vi "GetObjectID.vi"(0 "reference in":refnum<class "G#RemoteProxy.lvclass">, 5 "error in (no error)":errorcluster) -> (14 "reference out":refnum<class "G#RemoteProxy.lvclass">, 15 "object ID":u32 format="%x", 19 "error out":errorcluster)   [LabVIEW 2017, in "G#RemoteProxy.lvclass"]
doc: "Returns the unique object ID for the specified object."
uses:
  G#RemoteProxy.lvclass
  G#Object/G#Object.lvclass
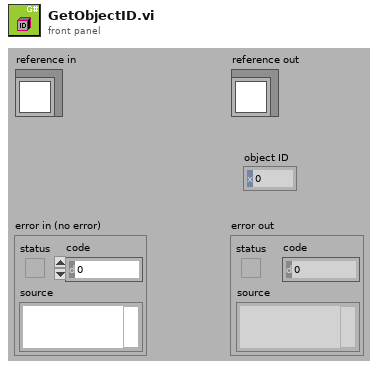
[diagram p1: front panel]
types:
  T1 = typedef "G#RemoteProxy.lvclass/ObjectAttributesProxy.ctl" = cluster{"class hierarchy":T2[], "class name":string, "lvlib hierarchy":string[], "full class name":string, "id":u32, "owner":string, "RemoteRef":refnum<class "G#Object.lvclass">, "object name":string, "attributes":variant[], "connection ID":refnum<k5>, "address":u32, "occurrence":refnum<k4>, "ProxyClassRef":refnum<class "G#RemoteProxy.lvclass">, "InMemory?":bool, "ToString":string}
  T2 = typedef "G#Object.lvclass/G#Object_ClassHierarchy.ctl" = cluster{"ClassName":string, "FullClassName":string, "ClassPath":path, "IsLeaf":bool}
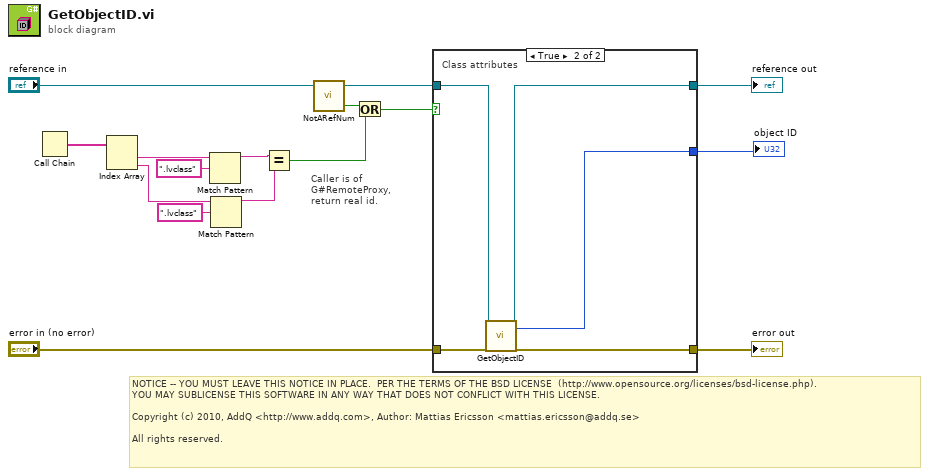
[diagram p0: block diagram]
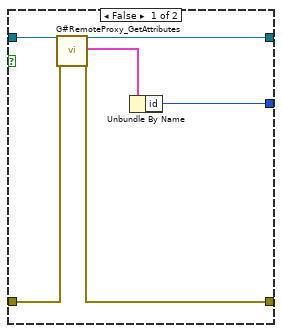
[diagram p2: hidden frame]
diagram:
  # "Caller is of\nG#RemoteProxy,\nreturn real id."
  # "NOTICE -- YOU MUST LEAVE THIS NOTICE IN PLACE.  PER THE TERMS OF THE BSD LICENSE  (http://www.opensource.org/licenses/bsd-license.php).\nYOU MAY SUBLICENSE THIS SOFTWARE IN ANY WAY THAT DOES NOT CONFLICT WITH THIS LICENSE.\n\nCopyright (c) 2010, AddQ <http://www.addq.com>, Author: Mattias Ericsson <mattias.ericsson@addq.se>\n\nAll rights reserved."
  n1 = Call Chain() -> (call chain=w10:string[])
  n2 = Index Array(array=w10) -> (element #1=w9:string, element #2=w6:string)  [unwired: 2 in]
  n3 = Match Pattern(string=w9, regular expression=".lvclass") -> (before substring=w5:string)  [unwired: 1 in, 3 out]
  n4 = Match Pattern(string=w6, regular expression=".lvclass") -> (before substring=w4:string)  [unwired: 1 in, 3 out]
  n5 = Equal?(x=w5, y=w4) -> (x = y?=w2:bool)
  n6 = call-dynamic "NotARefNum.vi"("reference in"="reference in") -> ("not a refnum?"=w3:bool, "reference out"=w12:refnum<class "G#RemoteProxy.lvclass">)  [unwired: 1 in]
  n7 = Or(x=w3, y=w2) -> (x .or. y?=w1:bool)
  n8 = case shown="True" w1 {
    tunnel: [w22 w24] -> w16
    tunnel: "error in (no error)" -> [w21 w27]
    tunnel: [w20 w26] -> w14
    tunnel: [w18 w23] -> w13
    tunnel: w12 -> [w17 w25]
    frame False {
      n9 = call "G#RemoteProxy_GetAttributes.vi"("reference in"=w17, "error in (no error)"=w21) -> ("reference out"=w22:refnum<class "G#RemoteProxy.lvclass">, "attributes"=w19:T1, "error out"=w20:errorcluster)  [unwired: 14 in, 1 out]
      n10 = Unbundle By Name(w19) -> ("id"=w18:u32)
    }
    frame True {
      # "Class attributes"
      n11 = call-parent "GetObjectID.vi"("reference in"=w25, "error in (no error)"=w27) -> ("reference out"=w24:refnum<class "G#RemoteProxy.lvclass">, "object ID"=w23:u32, "error out"=w26:errorcluster)  [unwired: 15 in]
    }
  }
  "error out" <- w14
  "reference out" <- w16
  "object ID" <- w13
